vi "Actor Destroy.vi"(11 "Actor Destroy in":refnum<class "Actor Destroy.lvclass">) -> (3 "Actor Destroy out":refnum<class "Actor Destroy.lvclass">)   [LabVIEW 2021, in "Actor Destroy.lvlib" / "Actor Destroy.lvclass"]
uses:
  Actor Destroy.lvclass
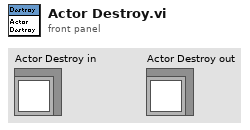
[diagram p1: front panel]
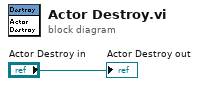
[diagram p0: block diagram]
diagram:
  "Actor Destroy out" <- "Actor Destroy in"
